vi "CS_cRIO-PB_DP-Master_ReadWrite.vi"(0 "FPGA VI Reference":T2, 2 "Mode":T1(ring), 5 "Slave":i8, 7 "Data":u8[](array[numeric]) format="%.0x", 11 "Error":errorcluster) -> (4 "FPGA VI Reference out":T2, 8 "Data out":u8[](array[numeric]) format="%.0x", 10 "Status":u8 format="%.0x", 15 "Error out":errorcluster)   [LabVIEW 2013, in "dynamic profibus.lvlib"]
uses:
  dynamic profibus.lvlib
  <vilib>/rvi/interface/nirviReadWriteControl/nirviReadWriteControl.xnode
  fpga reference.ctl
  <vilib>/rvi/errors/niLvFpgaAdjustHostInterfaceError.vi
  <vilib>/rvi/interface/Simulation/niFpgaSimulationCallBeginRW.vi
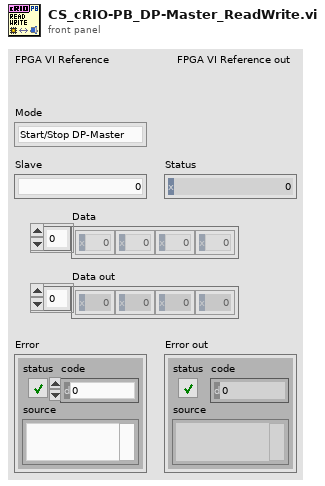
[diagram p1: front panel]
types:
  T1 = enum16{"Start/Stop DP-Master", "Get Input Data", "Set Output Data", "Get Output Data", "Get Diagnostic Data", "Read/Write Data", "Read Diagnostic Data", "Get DPV1 Data", "Set DPV1 Data", "Read/Write DPV1 Data"}
  T2 = typedef "dynamic profibus.lvlib/fpga reference.ctl" = refnum<k20>
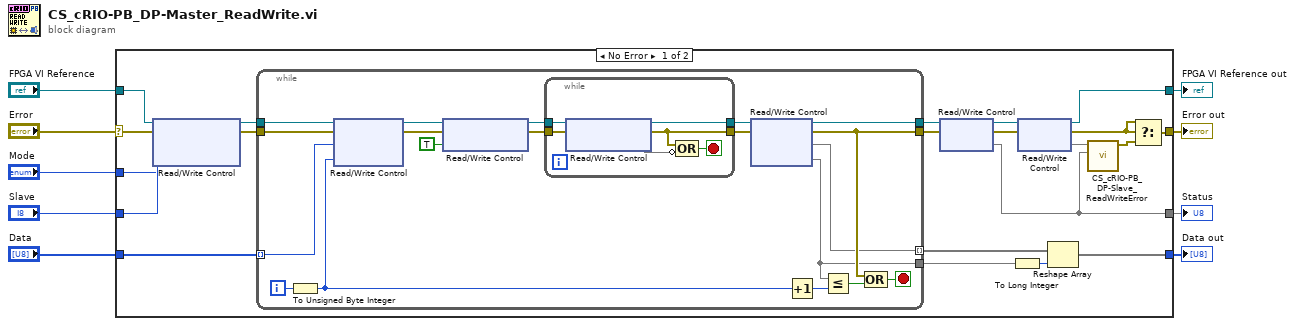
[diagram p0: block diagram]
diagram:
  n1 = case shown="No Error" "Error" {
    selector: "Error" -> [w30 w58]
    tunnel: "FPGA VI Reference" -> [w29 w57]
    tunnel: "Slave" -> [w28 _]
    tunnel: [w23 w58] -> w6
    tunnel: [w24 w57] -> w5
    tunnel: [w12 _] -> w4
    tunnel: "Data" -> [w18 w56]
    tunnel: [w15 w56] -> w2
    tunnel: "Mode" -> [w10 _]
    frame No Error {
      n2 = xnode "Read/Write Control"("FPGA VI Reference In"=w29, "error in"=w30, "Mode"=w10, "Slave/Service"=w28) -> ("FPGA VI Reference Out"=w19:T2, "error out"=w20:errorcluster)
      n3 = while {
        tunnel: w19 -> [w49]
        tunnel: [w41] -> w21
        tunnel: w20 -> [w40]
        tunnel: w18 -> [w38] mode=indexing
        tunnel: [w37] -> w22
        tunnel: [w32] -> w16
        tunnel: [w31] -> w14 mode=indexing
        i -> [w36]
        stop <- w42 stop-if-true
        n4 = To Unsigned Byte Integer(number=w36) -> (unsigned 8bit integer=w33:u8)
        n5 = xnode "Read/Write Control"("FPGA VI Reference In"=w49, "error in"=w40, "SetData"=w38, "ByteIndex"=w33) -> ("FPGA VI Reference Out"=w48:T2, "error out"=w47:errorcluster)
        n6 = xnode "Read/Write Control"("FPGA VI Reference In"=w48, "error in"=w47, "HostRequest"=TRUE ("GetData")) -> ("FPGA VI Reference Out"=w45:T2, "error out"=w46:errorcluster)
        n7 = while {
          tunnel: w46 -> [w55]
          tunnel: w45 -> [w51]
          tunnel: [w52] -> w44
          tunnel: [w50] -> w43
          stop <- w53 stop-if-true
          n8 = xnode "Read/Write Control"("FPGA VI Reference In"=w51, "error in"=w55) -> ("FPGA VI Reference Out"=w50:T2, "error out"=w52:errorcluster, "HostRequest"=w54)
          n9 = Compound Arithmetic op=OR(w52, invert w54) -> (w53:bool)
        }
        n10 = xnode "Read/Write Control"("FPGA VI Reference In"=w43, "error in"=w44) -> ("FPGA VI Reference Out"=w37:T2, "error out"=w41:errorcluster, "GetData"=w31, "DataLen"=w32)
        n11 = Increment(x=w33) -> (x+1=w35:u8)
        n12 = Less Or Equal?(x=w32, y=w35) -> (x <= y?=w34:bool)
        n13 = Compound Arithmetic op=OR(w41, w34) -> (w42:bool)
      }
      n14 = xnode "Read/Write Control"("FPGA VI Reference In"=w22, "error in"=w21) -> ("FPGA VI Reference Out"=w25:T2, "error out"=w26:errorcluster, "Status"=w12)
      n15 = To Long Integer(number=w16) -> (32bit integer=w17:i32)
      n16 = xnode "Read/Write Control"("FPGA VI Reference In"=w25, "error in"=w26) -> ("FPGA VI Reference Out"=w24:T2, "error out"=w27:errorcluster, "Error"=w13)
      n17 = Reshape Array(w14, w17) -> (w15:void[])
      n18 = call "CS_cRIO-PB_DP-Slave_ReadWriteError.vi"("Error"=w13, "Status"=w12) -> ("Error out"=w11:errorcluster)  [unwired: 7 in]
      n19 = Select(t=w27, s=w27, f=w11) -> (s? t:f=w23:errorcluster)
    }
    frame Error {
    }
  }
  "Error out" <- w6
  "FPGA VI Reference out" <- w5
  "Status" <- w4
  "Data out" <- w2
